vi "Read PID Params.vi"(8 "error in (no error)":errorcluster, 11 "TE Cooler in":refnum<class "TE Cooler.lvclass">) -> (0 "error out":errorcluster, 2 "PID Params":cluster{"P":dbl, "I":dbl, "D":dbl}={"P"=1.0, "I"=0.75, "D"=0.0}, 3 "TE Cooler out":refnum<class "TE Cooler.lvclass">)   [LabVIEW 2015, in "TE Cooler.lvlib" / "TE Cooler.lvclass"]
uses:
  TE Cooler.lvclass
  TE Cooler.lvclass/TE Cooler.ctl
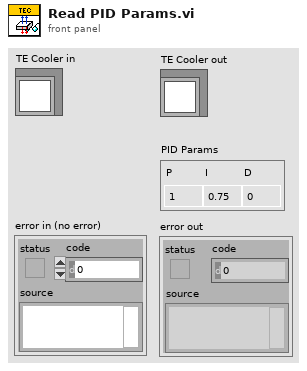
[diagram p1: front panel]
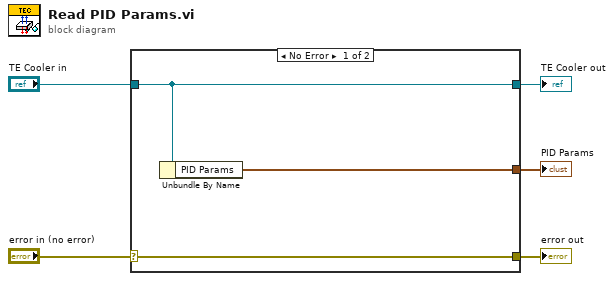
[diagram p0: block diagram]
diagram:
  n1 = case shown="No Error" "error in (no error)" {
    selector: "error in (no error)" -> [w8 w9]
    tunnel: [w8 w9] -> w4
    tunnel: [w7 w10] -> w2
    tunnel: "TE Cooler in" -> [w7 w10]
    tunnel: [w6 _] -> w1
    frame No Error {
      n2 = Unbundle By Name(w7) -> ("PID Params"=w6:cluster{"P":dbl, "I":dbl, "D":dbl})
    }
    frame Error {
    }
  }
  "error out" <- w4
  "TE Cooler out" <- w2
  "PID Params" <- w1
